vi "Color.vi"(11 "BGK Color":T1 {"alpha" scale=0.0..255.0}) -> (3 ".NET Refnum out":refnum<k24>)   [LabVIEW 2014, in "XMSChart.xctl"]
uses:
  XMSChart.xctl
  System.Drawing
  Controls/Color.ctl
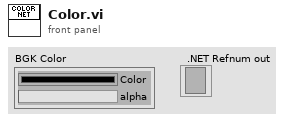
[diagram p1: front panel]
types:
  T1 = typedef "XMSChart.xctl/Color.ctl" = cluster{"Color":u32, "alpha":u8}
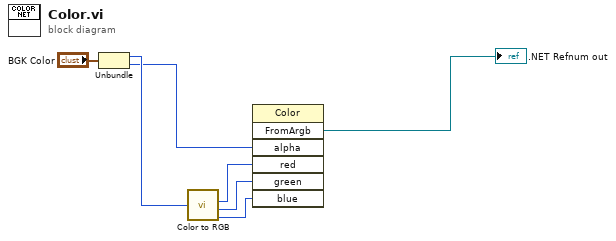
[diagram p0: block diagram]
diagram:
  n1 = Unbundle("BGK Color") -> ("Color"=w2:u32, "alpha"=w1:u8)
  n2 = call <vilib>:"Color to RGB.vi"("Color"=w2) -> ("R"=w4:u8, "G"=w5:u8, "B"=w6:u8)  [unwired: 1 out]
  n3 = invoke class="Color" method="FromArgb"("alpha"=w1, "red"=w4, "green"=w5, "blue"=w6) -> ("FromArgb"=→".NET Refnum out":refnum<k24>)  [unwired: 3 in, 6 out]
